vi "BRig_dataLC_Selection_PreR_Block_l2.vi"() -> (2 "output_Selection_PreR_Block_l2":i32)   [LabVIEW 2014]
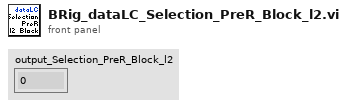
[diagram p1: front panel]
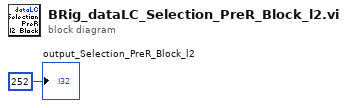
[diagram p0: block diagram]
diagram:
  "output_Selection_PreR_Block_l2" <- 252 ("output_iBlock")
